vi "Instantiate Container.vi"(8 "error in (no error)":errorcluster) -> (0 "error out":errorcluster, 3 "Container base out":refnum<class "Container base.lvclass">)   [LabVIEW 2016, in "Container base.lvclass"]
uses:
  Container base.lvclass
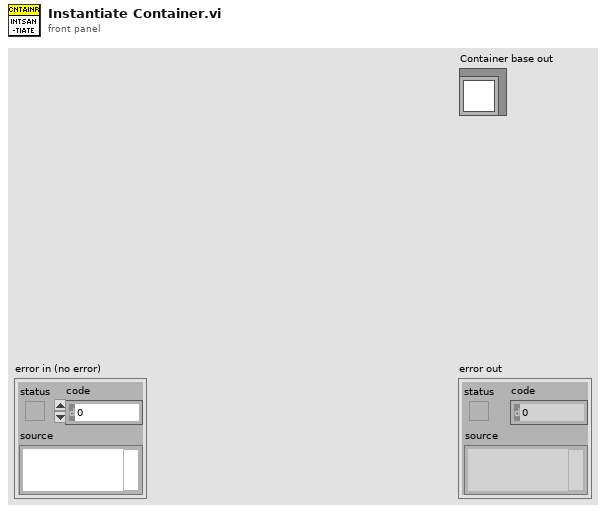
[diagram p1: front panel]
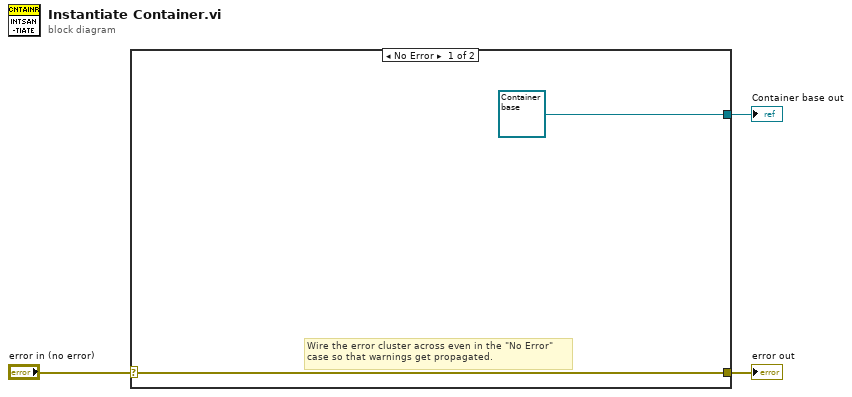
[diagram p0: block diagram]
diagram:
  n1 = case shown="No Error" "error in (no error)" {
    selector: "error in (no error)" -> [w5 w6]
    tunnel: [w5 w6] -> w2
    tunnel: [refnum<class "Container base.lvclass"> refnum ("Container base out") _] -> w1
    frame No Error {
      # "Wire the error cluster across even in the \"No Error\"\ncase so that warnings get propagated."
    }
    frame Error {
    }
  }
  "error out" <- w2
  "Container base out" <- w1
